vi "CreateActionQueues.vi"(8 "Error In":errorcluster) -> (0 "Error Out":errorcluster, 3 "Action Queues":T1)   [LabVIEW 2012]
uses:
  ActionQueues.ctl
  UIActionQueueElement.ctl
  UIAction.ctl
  HardwareActionQueueElement.ctl
  HardwareAction.ctl
  ExperimentActionQueueElement.ctl
  ExperimentAction.ctl
  AlarmQueueElement.ctl
  AlarmAction.ctl
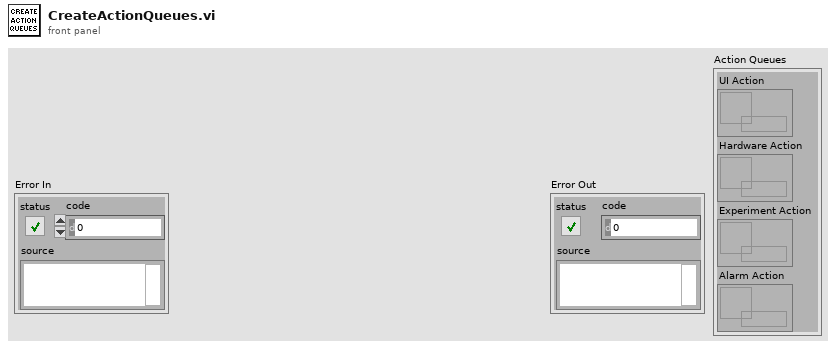
[diagram p1: front panel]
types:
  T1 = typedef "ActionQueues.ctl" = cluster{"UI Action":refnum<queue>, "Hardware Action":refnum<queue>, "Experiment Action":refnum<queue>, "Alarm Action":refnum<queue>}
  T2 = typedef "AlarmQueueElement.ctl" = cluster{"Action":T3, "Data":variant}
  T3 = typedef "AlarmAction.ctl" = enum16{"Initialize", "Load", "Check", "Shutdown"}
  T4 = typedef "ExperimentActionQueueElement.ctl" = cluster{"Action":T5, "Data":variant}
  T5 = typedef "ExperimentAction.ctl" = enum16{"Initialize", "Create", "Read", "Load", "Start", "Run", "Stop", "Save", "Shutdown"}
  T6 = typedef "HardwareActionQueueElement.ctl" = cluster{"Action":T7, "Data":variant}
  T7 = typedef "HardwareAction.ctl" = enum16{"Initialize", "Collect", "Shutdown"}
  T8 = typedef "UIActionQueueElement.ctl" = cluster{"Action":T9, "Data":variant}
  T9 = typedef "UIAction.ctl" = enum16{"Initalize", "Create Experiment", "Created", "Read Experiment Controls", "Read Alarm Controls", "Loaded", "Save Experiment", "Saved", "Write Experiment Controls", "Read Experiment", "Read", "Start Experiment", "Started", "Stop Experiment", "Stopped", "Close Experiment", "Closed", "SRIM", "Error", "Shutdown"}
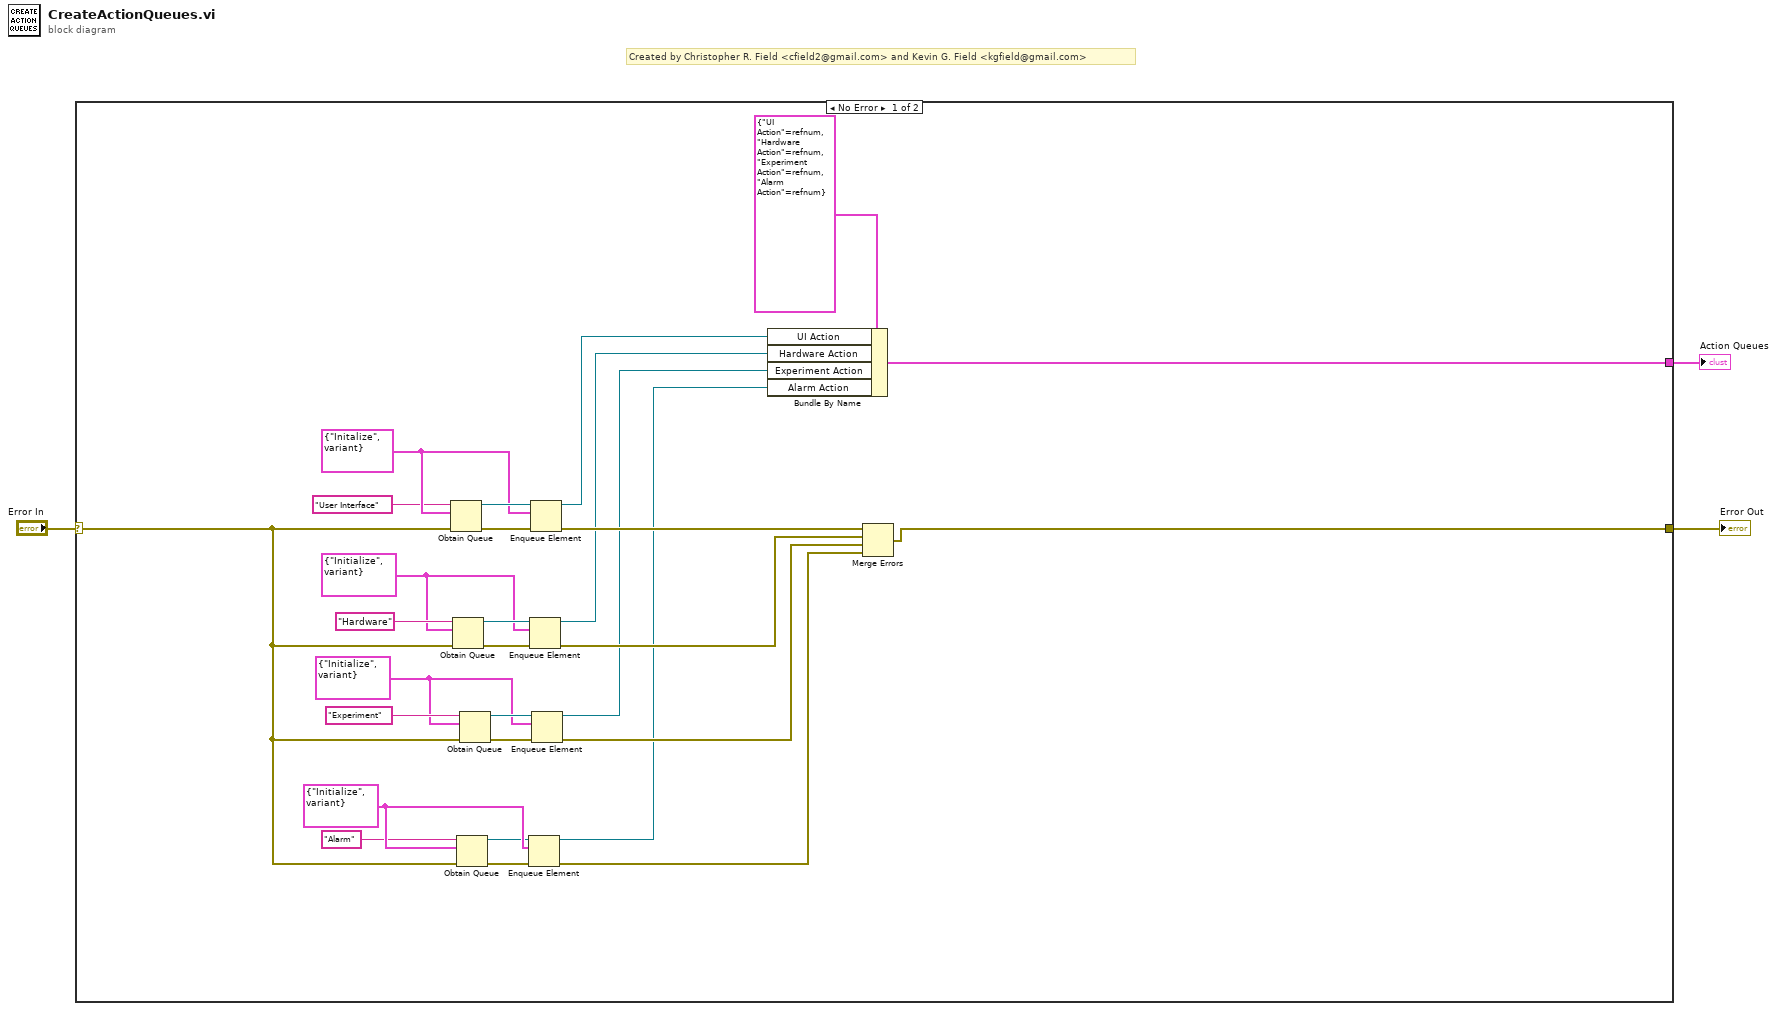
[diagram p0: block diagram]
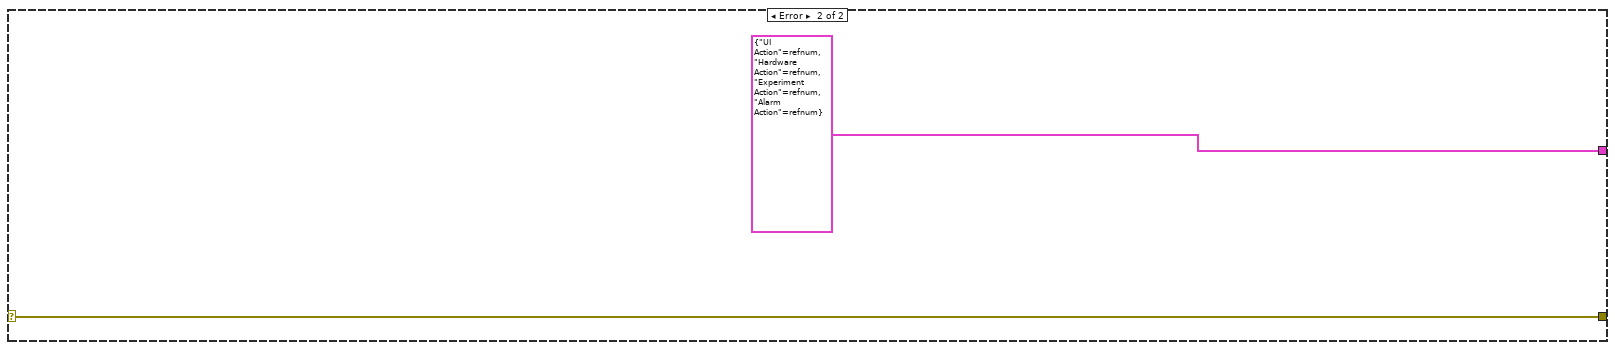
[diagram p2: hidden frame]
diagram:
  # "Created by Christopher R. Field <cfield2@gmail.com> and Kevin G. Field <kgfield@gmail.com>"
  n1 = case shown="No Error" "Error In" {
    selector: "Error In" -> [w5 w33]
    tunnel: [w25 w33] -> w2
    tunnel: [w17 T1 {"UI Action"=refnum, "Hardware Action"=refnum, "Experiment Action"=refnum, "Alarm Action"=refnum} ("Message Queues")] -> w1
    frame No Error {
      w10 = T2 {"Action"=enum."Initialize", "Data"=variant} ("Alarm Queue Element")
      w13 = T4 {"Action"=enum."Initialize", "Data"=variant} ("Experiment Action Queue Element")
      w21 = T6 {"Action"=enum."Initialize", "Data"=variant} ("Hardware Queue Element")
      w24 = T8 {"Action"=enum."Initalize", "Data"=variant} ("User Interface Queue Element")
      n2 = Obtain Queue(name (unnamed)="User Interface", element data type=w24, error in (no error)=w5) -> (queue out=w30:refnum<queue>, error out=w31:errorcluster)  [unwired: 2 in, 1 out]
      n3 = Obtain Queue(name (unnamed)="Hardware", element data type=w21, error in (no error)=w5) -> (queue out=w28:refnum<queue>, error out=w29:errorcluster)  [unwired: 2 in, 1 out]
      n4 = Obtain Queue(name (unnamed)="Alarm", element data type=w10, error in (no error)=w5) -> (queue out=w9:refnum<queue>, error out=w7:errorcluster)  [unwired: 2 in, 1 out]
      n5 = Obtain Queue(name (unnamed)="Experiment", element data type=w13, error in (no error)=w5) -> (queue out=w15:refnum<queue>, error out=w14:errorcluster)  [unwired: 2 in, 1 out]
      n6 = Enqueue Element(queue=w9, element=w10, error in (no error)=w7) -> (queue out=w4:refnum<queue>, error out=w6:errorcluster)  [unwired: 1 in, 1 out]
      n7 = Enqueue Element(queue=w28, element=w21, error in (no error)=w29) -> (queue out=w18:refnum<queue>, error out=w26:errorcluster)  [unwired: 1 in, 1 out]
      n8 = Enqueue Element(queue=w30, element=w24, error in (no error)=w31) -> (queue out=w19:refnum<queue>, error out=w27:errorcluster)  [unwired: 1 in, 1 out]
      n9 = Enqueue Element(queue=w15, element=w13, error in (no error)=w14) -> (queue out=w11:refnum<queue>, error out=w12:errorcluster)  [unwired: 1 in, 1 out]
      n10 = Bundle By Name(cluster=T1 {"UI Action"=refnum, "Hardware Action"=refnum, "Experiment Action"=refnum, "Alarm Action"=refnum} ("Message Queues"), "UI Action"=w19, "Hardware Action"=w18, "Experiment Action"=w11, "Alarm Action"=w4) -> (w17:T1)
      n11 = Merge Errors(w27, w26, w12, w6) -> (w25:errorcluster)
    }
    frame Error {
    }
  }
  "Error Out" <- w2
  "Action Queues" <- w1
